vi "List Managers.vi"(10 "Include Cache? (F)":bool, 11 "ConfigManager in":refnum<class "ConfigManager.lvclass">) -> (2 "List":refnum<class "ConfigManager.lvclass">[](array[class]), 3 "ConfigManager out":refnum<class "ConfigManager.lvclass">)   [LabVIEW 2013, in "CfgManager.lvlib" / "ConfigManager.lvclass"]
uses:
  ConfigManager.lvclass
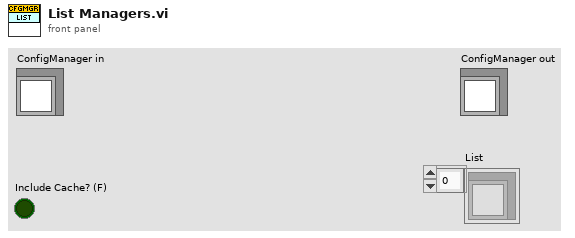
[diagram p1: front panel]
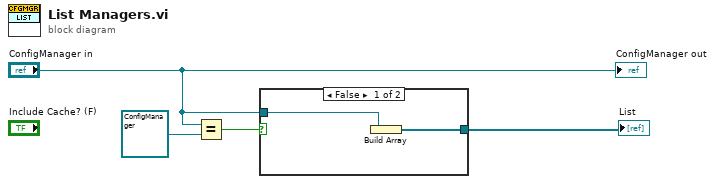
[diagram p0: block diagram]
diagram:
  n1 = Equal?(x="ConfigManager in", y=refnum<class "ConfigManager.lvclass"> refnum) -> (x = y?=w3:bool)
  n2 = case shown="False" w3 {
    tunnel: "ConfigManager in" -> [w6 _]
    tunnel: [w5 _] -> w1
    frame False {
      n3 = Build Array(w6) -> (w5:refnum<class "ConfigManager.lvclass">[])
    }
    frame True {
    }
  }
  "List" <- w1
  "ConfigManager out" <- "ConfigManager in"
